vi "Read Attributes.vi"(11 "PF Commands Msg":refnum<class "PF Commands Msg.lvclass">) -> (2 "Payload":cluster{"Run":bool, "Setpoint":dbl})   [LabVIEW 2019, in "Platform.lvlib" / "PF Commands Msg.lvclass"]
uses:
  PF Commands Msg.lvclass
  PF Commands Msg.lvclass/PF Commands Msg.ctl
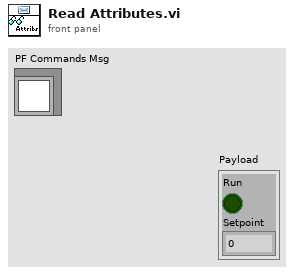
[diagram p1: front panel]
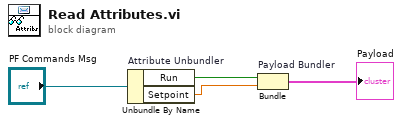
[diagram p0: block diagram]
diagram:
  n1 = Unbundle By Name "Attribute Unbundler"("PF Commands Msg") -> ("Run"=w2:bool, "Setpoint"=w1:dbl)
  n2 = Bundle "Payload Bundler"("Run"=w2, "Setpoint"=w1) -> (→"Payload":cluster{"Run":bool, "Setpoint":dbl})  [unwired: 1 in]
